vi "Benchmark_GetName.vi"() -> ()   [LabVIEW 2013]
uses:
  source/TypeDescriptor/TypeDescriptor_GetName.vi
  source/TypeDescriptor/TypeDescriptor_GetPString.vi
  source/TypeDescriptor/TypeDescriptor_SetName.vi
  source/Variant/OpenVariant.lvlib
panel:
  out "Array":string[](array[string])
  out "Waveform Chart":dbl(graph)
  out "execution time per call":dbl
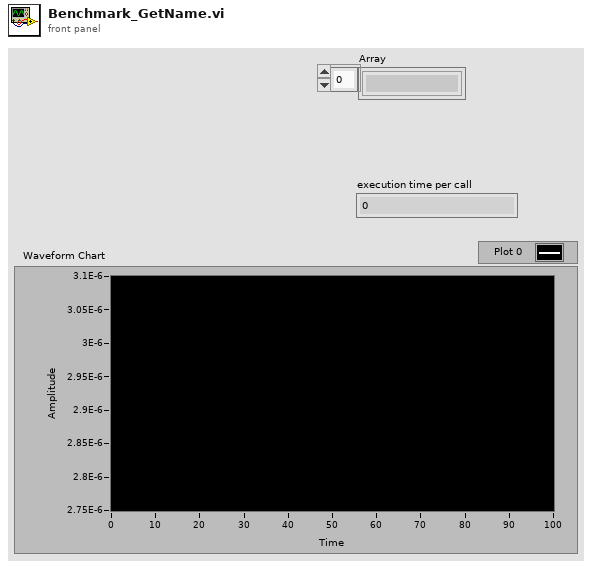
[diagram p1: front panel]
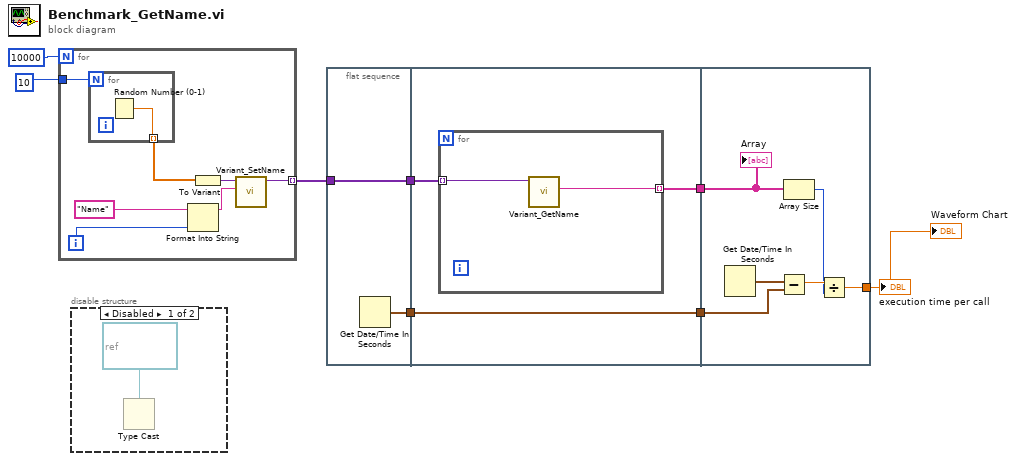
[diagram p0: block diagram]
diagram:
  n1 = for {
    N: 10000 -> [_]
    tunnel: [w12] -> w7 mode=indexing
    tunnel: 10 -> [w9]
    i -> [w11]
    n2 = for {
      N: w9 -> [_]
      tunnel: [w16] -> w10 mode=indexing
      n3 = Random Number (0-1)() -> (number: 0 to 1=w16:dbl)
    }
    n4 = Format Into String(initial string="Name", w11) -> (resulting string=w13:string)  [unwired: 2 in, 1 out]
    n5 = To Variant(anything=w10) -> (Variant=w14:variant)
    n6 = call "Variant_SetName.vi"("Name"=w13, "Variant"=w14) -> ("Named Variant"=w12:variant)  [unwired: 9 in]
  }
  n7 = disable-structure shown="Disabled" {
    frame Disabled {
      n8 = Type Cast(type=refnum<queue> refnum ("queue out")) -> ()  [unwired: 1 in, 1 out]
    }
    frame Enabled {
    }
  }
  n9 = flat-sequence {
    tunnel: w7 -> [w19]
    tunnel: [w19] -> w6
    tunnel: [w18] -> w4
    tunnel: w6 -> [w22]
    tunnel: [w21] -> w5
    tunnel: w4 -> [w21]
    tunnel: [w20] -> w2
    tunnel: w5 -> [w29]
    tunnel: [w26] -> w3
    tunnel: w2 -> [w25]
    frame #0 {
      n10 = Get Date/Time In Seconds() -> (seconds since 1Jan1904=w18:timestamp)
    }
    frame #1 {
      n11 = for {
        tunnel: w22 -> [w24] mode=indexing
        tunnel: [w23] -> w20 mode=indexing
        n12 = call "Variant_GetName.vi"("Variant"=w24) -> ("Name"=w23:string)  [unwired: 8 in, 2 out]
      }
    }
    frame #2 {
      n13 = Get Date/Time In Seconds() -> (seconds since 1Jan1904=w30:timestamp)
      n14 = Subtract(x=w30, y=w29) -> (x-y=w28:dbl)
      n15 = Array Size(array=w25) -> (size(s)=w27:i32)
      n16 = Divide(x=w28, y=w27) -> (x/y=w26:dbl)
      "Array" <- w25
    }
  }
  "execution time per call" <- w3
  "Waveform Chart" <- w3
